vi "Turn_IMU_Abs.vi"(0 "Timeout (s)":dbl, 1 "Acceptable Error (Degrees)":dbl, 2 "Kp":dbl=0.05, 3 "Target (Degrees)":dbl) -> ()   [LabVIEW 2020]
uses:
  <vilib>/Rock Robotics/WPI/Utilities/WPI_GetSetVariantRefNum.vi
  <vilib>/Rock Robotics/WPI/ThirdParty/Phoenix-LabVIEW/Pigeon IMU/CTRE_PigeonIMU_GetYPR.vi
  <vilib>/Rock Robotics/WPI/RobotDrive/WPI_RobotDriveArcadeDrive_Standard(NoSaturation).vi
panel:
  out "Times Target Successful":dbl
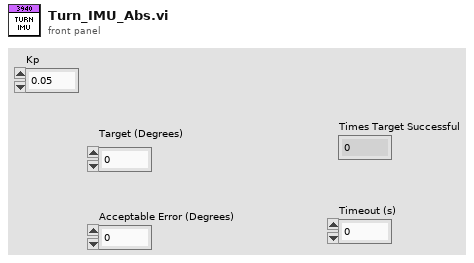
[diagram p1: front panel]
types:
  T1 = typedef "CTRE_PigeonIMU_DeviceRef.ctl" = cluster{"DeviceStatus":errorcluster, "Device Number":u8, "Type":T2, "Device ID":u32, "Handle":u64, "UsageFrame":u32, "Library Path":path}
  T2 = typedef "CTRE_PigeonIMU_ConnectionType.ctl" = u32
  T3 = typedef "WPI_RobotDriveDevRef.ctl" = cluster{"DevStatus":errorcluster, "Motors[]":T4[], "Square Inputs":bool, "Max Output":dbl}
  T4 = typedef "WPI_MotorControlDeviceRef.ctl" = cluster{"DeviceStatus":errorcluster, "Type":T5, "PWM":cluster{"PWM Channel":T6, "DeadBand":T7}, "CAN":cluster{"Device Number":u8, "SetOutput VI Ref":variant, "GetOutput VI Ref":variant, "Enable VI Ref":variant, "Disable VI Ref":variant, "Data":variant}, "Invert":bool, "DIO PWM":cluster{"PWM \"Enable\" Channel":T6, "DIOChannel":T8, "PWM Rate":dbl}}
  T5 = typedef "WPI_MotorControlType.ctl" = enum16{"PWM", "CAN", "DIO PWM"}
  T6 = typedef "FPGA_DIOPWMChannel.ctl" = enum8{"PWM 0", "PWM 1", "PWM 2", "PWM 3", "PWM 4", "PWM 5", "PWM 6", "PWM 7", "PWM 8", "PWM 9", "PWM MXP 0", "PWM MXP 1", "PWM MXP 2", "PWM MXP 3", "PWM MXP 4", "PWM MXP 5", "PWM MXP 6", "PWM MXP 7", "PWM MXP 8", "PWM MXP 9", "Invalid"}
  T7 = typedef "WPI_PWMDeadband.ctl" = cluster{"Name":string, "maxPositivePwm":i32, "minPositivePwm":i32, "centerPwm":i32, "maxNegativePwm":i32, "minNegativePwm":i32, "angularRange":u16}
  T8 = typedef "FPGA_DIOChannel.ctl" = enum8{"DIO 0", "DIO 1", "DIO 2", "DIO 3", "DIO 4", "DIO 5", "DIO 6", "DIO 7", "DIO 8", "DIO 9", "DIO MXP 0", "DIO MXP 1", "DIO MXP 2", "DIO MXP 3", "DIO MXP 4", "DIO MXP 5", "DIO MXP 6", "DIO MXP 7", "DIO MXP 8", "DIO MXP 9", "DIO MXP 10", "DIO MXP 11", "DIO MXP 12", "DIO MXP 13", "DIO MXP 14", "DIO MXP 15", "SPI Port CS1", "SPI Port CS2", "SPI Port CS3", "SPI Port MISO", "SPI Port MOSI", "Invalid"}
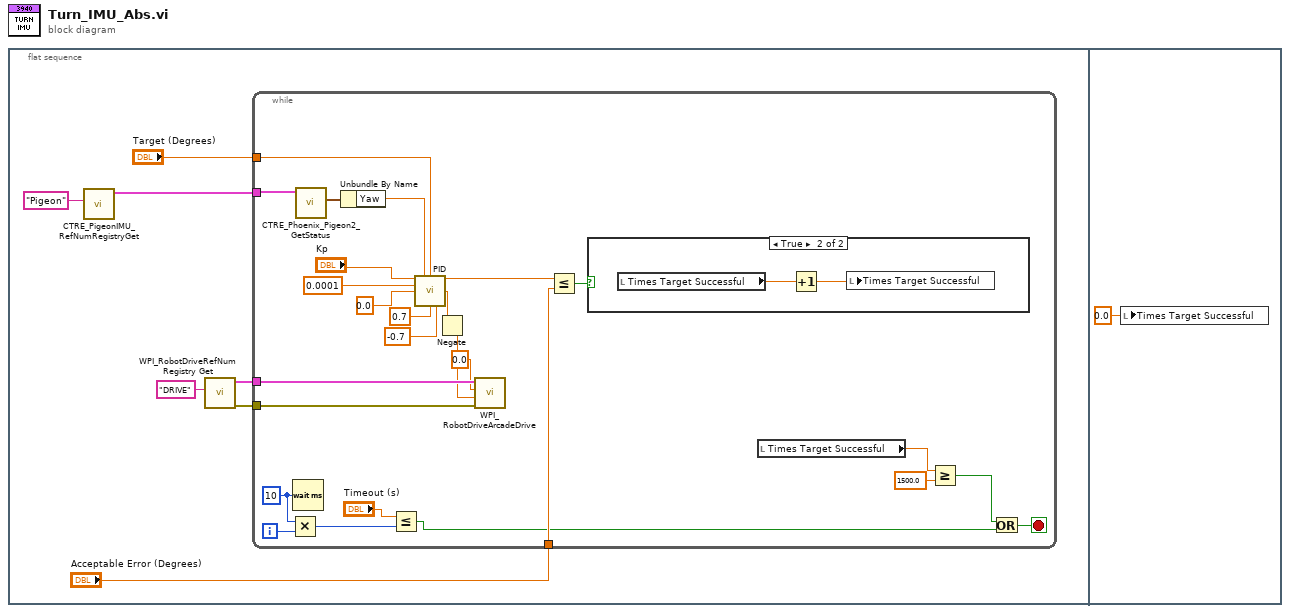
[diagram p0: block diagram]
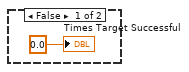
[diagram p2: hidden frame]
diagram:
  n1 = flat-sequence {
    frame #0 {
      n2 = call <vilib>:"CTRE_PigeonIMU_RefNumRegistryGet.vi"("refnum name"="Pigeon") -> ("PigeonIMUDevRef"=w1:T1)  [unwired: 9 in, 1 out]
      n3 = call <vilib>:"WPI_RobotDriveRefNum Registry Get.vi"("refnum name"="DRIVE") -> ("error out"=w3:errorcluster, "RobotDriveDevRef"=w4:T3)  [unwired: 9 in]
      n4 = while {
        tunnel: w1 -> [w32]
        tunnel: "Target (Degrees)" -> [w9]
        tunnel: "Acceptable Error (Degrees)" -> [w28]
        tunnel: w4 -> [w15]
        tunnel: w3 -> [w14]
        i -> [w24]
        stop <- w20 stop-if-true
        w23 = u32 10 ("milliseconds to wait")
        n5 = Multiply(x=w23, y=w24) -> (x*y=w22:u32)
        n6 = Wait (ms)(milliseconds to wait=w23) -> ()  [unwired: 1 out]
        n7 = call-poly <vilib>:"CTRE_Phoenix_Pigeon2_GetStatus.vi"("PigeonIMUDevRef"=w32) -> ("Yaw Pitch Roll"=w33:cluster{"Yaw":dbl, "Pitch":dbl, "Roll":dbl})  [unwired: 8 in, 2 out]
        n8 = Unbundle By Name(w33) -> ("Yaw"=w11:dbl)
        n9 = Less Or Equal?(x="Timeout (s)", y=w22) -> (x <= y?=w18:bool)
        n10 = call "PID.vi"("Kp"="Kp", "Process Variable"=w11, "Goal"=w9, "Ki"=0.0001, "Kd"=0.0, "Max Ouput"=0.7, "Min Output"=-0.7) -> ("Current Error"=w29:dbl, "Command"=w13:dbl)  [unwired: 6 in, 1 out]
        n11 = Negate(x=w13) -> (-x=w10:dbl)
        n12 = call-poly <vilib>:"WPI_RobotDriveArcadeDrive.vi"("error in (no error)"=w14, "Y axis value"=w10, "X axis value"=0.0, "RobotDriveDevRef"=w15) -> ()  [unwired: 5 in, 3 out]
        n13 = Less Or Equal?(x=w29, y=w28) -> (x <= y?=w27:bool)
        n14 = case shown="True" w27 {
          frame False {
            "Times Target Successful" <- 0.0
          }
          frame True {
            n15 = local read "Times Target Successful"() -> (w36:dbl)
            n16 = Increment(x=w36) -> (x+1=w35:dbl)
            n17 = local write "Times Target Successful"(w35) -> ()
          }
        }
        n18 = local read "Times Target Successful"() -> (w25:dbl)
        n19 = Greater Or Equal?(x=w25, y=1500.0) -> (x >= y?=w19:bool)
        n20 = Or(x=w19, y=w18) -> (x .or. y?=w20:bool)
      }
    }
    frame #1 {
      n21 = local write "Times Target Successful"(0.0 ("Times Target Successful")) -> ()
    }
  }
